vi "ajuda.vi"() -> ()   [LabVIEW 2018]
panel:
  in  "Close":bool
  in  "Adicionar 4":bool
  in  "Adicionar 3":bool
  in  "Adicionar 2":bool
  in  "Adicionar":bool
  # "Menu de"
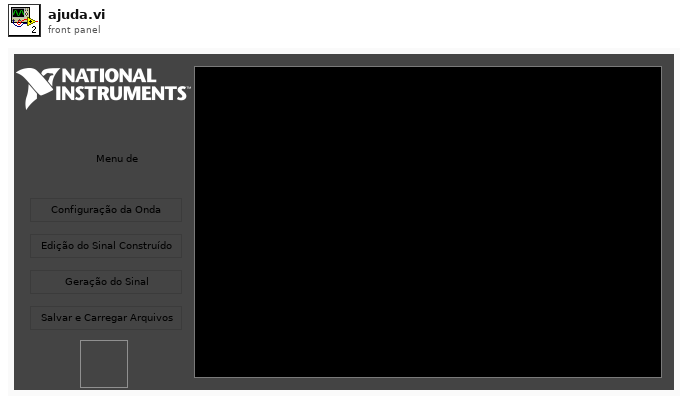
[diagram p1: front panel]
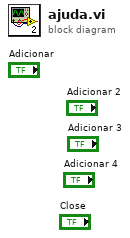
[diagram p0: block diagram]
diagram:
